vi "Conveyer Belt Set.vi"(1 "Conveyer Belt Information In":T1) -> (0 "Conveyer Belt Information Out":T1)   [LabVIEW 2012]
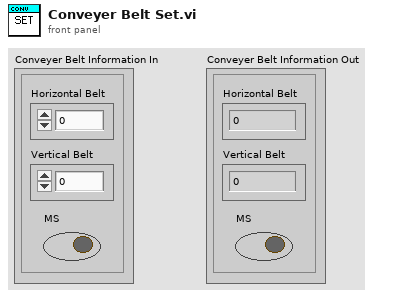
[diagram p1: front panel]
types:
  T1 = cluster{"Horizontal Belt":dbl, "Vertical Belt":dbl, "MS":bool}
  T2 = typedef "WPI_RelayValue.ctl" = enum16{"Off", "On", "Forward", "Reverse"}
  T3 = typedef "WPI_RelayDevRef.ctl" = cluster{"DevStatus":errorcluster, "Relay Channel":T4, "Digital Module":T5, "Relay Direction":T6}
  T4 = typedef "FPGA_DIORelayChannel.ctl" = enum8{"Relay 1", "Relay 2", "Relay 3", "Relay 4", "Relay 5", "Relay 6", "Relay 7", "Relay 8", "Invalid"}
  T5 = typedef "FPGA_TypedefDigitalModule.ctl" = enum16{"Digital Module 1", "Digital Module 2"}
  T6 = typedef "WPI_RelayDirection.ctl" = enum16{"Both directions", "Forward only", "Reverse only"}
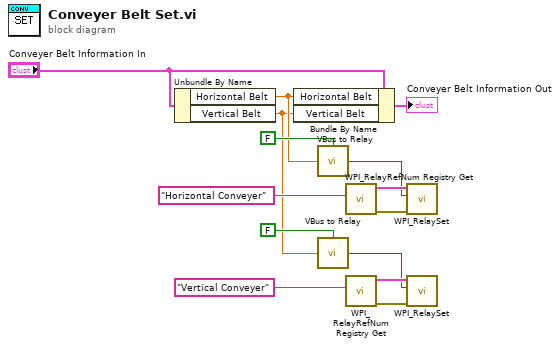
[diagram p0: block diagram]
diagram:
  n1 = Unbundle By Name("Conveyer Belt Information In") -> ("Horizontal Belt"=w2:dbl, "Vertical Belt"=w1:dbl)
  n2 = Bundle By Name(cluster="Conveyer Belt Information In", "Horizontal Belt"=w2, "Vertical Belt"=w1) -> (→"Conveyer Belt Information Out":T1)
  n3 = call "VBus to Relay.vi"("Invert Relay? (F)"=FALSE, "Motor VBus"=w2) -> ("RelayValue"=w6:T2)  [unwired: 2 in]
  n4 = call "VBus to Relay.vi"("Invert Relay? (F)"=FALSE, "Motor VBus"=w1) -> ("RelayValue"=w5:T2)  [unwired: 2 in]
  n5 = call <vilib>:"WPI_RelayRefNum Registry Get.vi"("refnum name"="Horizontal Conveyer") -> ("error out"=w12:errorcluster, "RelayDevRef"=w11:T3)  [unwired: 9 in]
  n6 = call <vilib>:"WPI_RelayRefNum Registry Get.vi"("refnum name"="Vertical Conveyer") -> ("error out"=w14:errorcluster, "RelayDevRef"=w13:T3)  [unwired: 9 in]
  n7 = call <vilib>:"WPI_RelaySet.vi"("error in (no error)"=w12, "RelayValue"=w6, "RelayDevRef"=w11) -> ()  [unwired: 7 in, 2 out]
  n8 = call <vilib>:"WPI_RelaySet.vi"("error in (no error)"=w14, "RelayValue"=w5, "RelayDevRef"=w13) -> ()  [unwired: 7 in, 2 out]
